vi "ARDRegression.vi"(8 "error in":errorcluster) -> (0 "error out":errorcluster, 3 "out":refnum<class "ARDRegression.lvclass">)   [LabVIEW 2020]
doc: "Bayesian ARD regression.\n\n Fit the weights of a regression model, using an ARD prior. The weights of\n the regression model are assumed to be in Gaussian distributions.\n Also estimate the parameters lambda (precisions of the distributions of the\n weights) and alpha (precision of the distribution of the noise).\n The estimation is done by an iterative procedures (Evidence Maximization)\n\n Read more in the :ref:`User Guide <bayesian_regression>`.\n\n Parameters\n ----------\n n_iter : int, default=300\n Maximum number of iterations.\n\n tol : float, default=1e-3\n Stop the algorithm if w has converged.\n\n alpha_1 : float, default=1e-6\n Hyper-parameter : shape parameter for the Gamma distribution prior\n over the alpha parameter.\n\n alpha_2 : float, default=1e-6\n Hyper-parameter : inverse scale parameter (rate parameter) for the\n Gamma distribution prior over the alpha parameter.\n\n lambda_1 : float, default=1e-6\n Hyper-parameter : shape parameter for the Gamma distribution prior\n over the lambda parameter.\n\n lambda_2 : float, default=1e-6\n Hyper-parameter : inverse scale parameter (rate parameter) for the\n Gamma distribution prior over the lambda parameter.\n\n compute_score : bool, default=False\n If True, compute the objective function at each step of the model.\n\n threshold_lambda : float, default=10 000\n threshold for removing (pruning) weights with high precision from\n the computation.\n\n fit_intercept : bool, default=True\n whether to calculate the intercept for this model. If set\n to false, no intercept will be used in calculations\n (i.e. data is expected to be centered).\n\n normalize : bool, default=False\n This parameter is ignored when ``fit_intercept`` is set to False.\n If True, the regressors X will be normalized before regression by\n subtracting the mean and dividing by the l2-norm.\n If you wish to standardize, please use\n :class:`~sklearn.preprocessing.StandardScaler` before calling ``fit``\n on an estimator with ``normalize=False``.\n\n copy_X : bool, default=True\n If True, X will be copied; else, it may be overwritten.\n\n verbose : bool, default=False\n Verbose mode when fitting the model.\n\n Attributes\n ----------\n coef_ : array-like of shape (n_features,)\n Coefficients of the regression model (mean of distribution)\n\n alpha_ : float\n estimated precision of the noise.\n\n lambda_ : array-like of shape (n_features,)\n estimated precisions of the weights.\n\n sigma_ : array-like of shape (n_features, n_features)\n estimated variance-covariance matrix of the weights\n\n scores_ : float\n if computed, value of the objective function (to be maximized)\n\n intercept_ : float\n Independent term in decision function. Set to 0.0 if\n ``fit_intercept = False``.\n\n X_offset_ : float\n If `normalize=True`, offset subtracted for centering data to a\n zero mean.\n\n X_scale_ : float\n If `normalize=True`, parameter used to scale data to a unit\n standard deviation.\n\n \nAvailable methods:\nGet Attributes\nGet Params\nSet Params"
uses:
  ARDRegression.lvclass
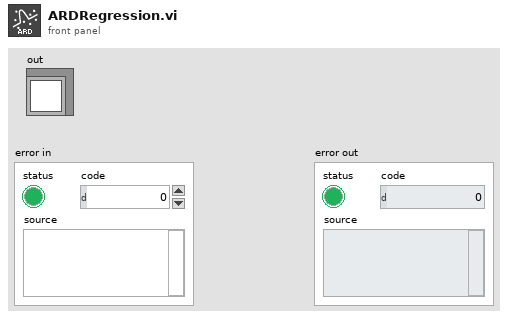
[diagram p1: front panel]
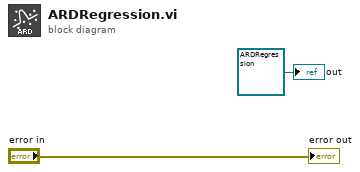
[diagram p0: block diagram]
diagram:
  "out" <- refnum<class "ARDRegression.lvclass"> refnum ("model")
  "error out" <- "error in"
